vi "Write VI Ref.vi"(8 "error in (no error)":errorcluster, 10 "VI Ref":refnum<vi>, 11 "TestEngineReference in":refnum<class "TestEngineReference.lvclass">) -> (0 "error out":errorcluster, 3 "TestEngineReference out":refnum<class "TestEngineReference.lvclass">)   [LabVIEW 2019, in "TestEngine.lvlib" / "TestEngineReference.lvclass"]
uses:
  TestEngineReference.lvclass
  TestEngineReference.lvclass/TestEngineReference.ctl
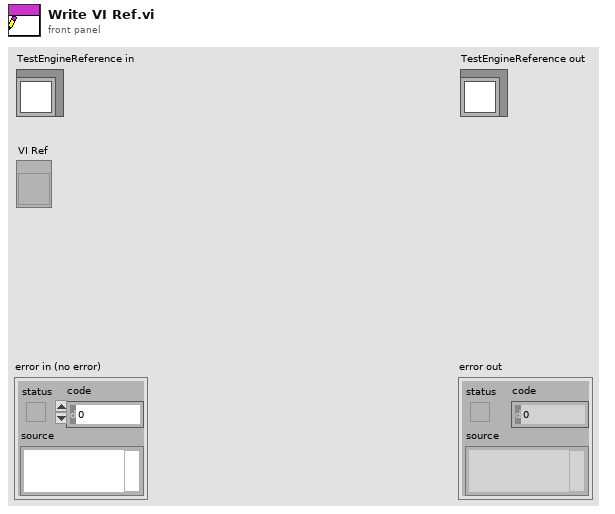
[diagram p1: front panel]
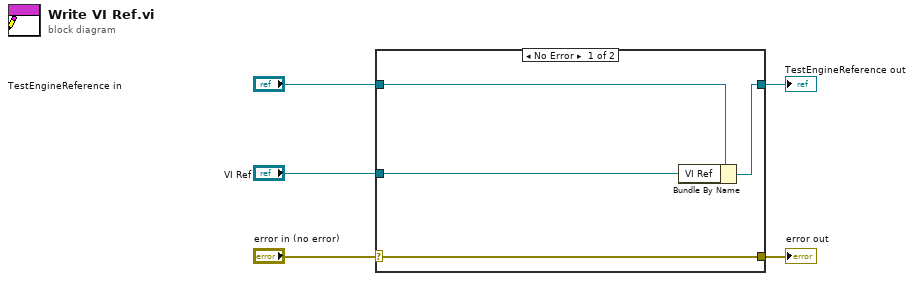
[diagram p0: block diagram]
diagram:
  n1 = case shown="No Error" "error in (no error)" {
    selector: "error in (no error)" -> [w9 w10]
    tunnel: [w9 w10] -> w4
    tunnel: [w7 w11] -> w2
    tunnel: "TestEngineReference in" -> [w8 w11]
    tunnel: "VI Ref" -> [w6 _]
    frame No Error {
      n2 = Bundle By Name(cluster=w8, "VI Ref"=w6) -> (w7:refnum<class "TestEngineReference.lvclass">)
    }
    frame Error {
    }
  }
  "error out" <- w4
  "TestEngineReference out" <- w2
